vi "全局1.vi"() -> ()   [LabVIEW 2016, in "数据传输系统-05.lvlib"]
panel:
  out "2086上传":bool caption="2086"
  out "固件版本":T1
  out "版本信息":string
  out "系统信息":u16[](array[numeric]) caption="校准点信息"
  in  "告警信息":T2
  out "配置文件队列名":T3
  out "校准信息改变时间":string
  in  "采配水关键参数":cluster{"配水时间":dbl, "沉淀时间":dbl, "清洗时间":dbl}
  in  "CODCr校准信息":T4
  in  "总氮校准信息":T4
  in  "总磷校准信息":T4
  in  "氨氮校准信息":T4
  in  "CODMn校准信息":T4
  out "校准信息改变":T5
  out "关键参数改变":T6
  in  "CODCr关键参数":T7
  in  "总氮关键参数":T7
  in  "总磷关键参数":T7
  in  "氨氮关键参数":T7
  in  "CODMn关键参数":T7
  out "读取各参数测量周期的值":u16[](array[numeric]) caption="读取试剂余量的值"
  out "读取试剂余量的值":u16[](array[numeric])
  out "软件自动重启":dbl
  out "与工控软件通信":bool
  in  "QN":string
  in  "命令编码CN":string
  in  "数据":string
  out "数据发送起始时间":timestamp format="%<%.3X\n%Y/%m/%d>T"
  out "数据接收超时指示灯":bool
  out "实时小时数据上传":bool
  out "核查数据上传":bool
  out "反控数据":bool caption="超标留样"
  in  "table元素":string
  out "超标留样":bool
  out "测量周期":bool
  out "运行模式":bool
  out "系统状态":bool
  out "读取报文首页显示":string
  out "发送报文首页显示":string
  out "通讯包字符串":string
  out "数据输出":string
  out "register values":u16[](array[numeric]) caption="读取寄存器的值"
  out "系统编码ST":string="21"
  in  "枚举":enum16{"返回请求应答", "上传数据", "返回执行结果"}(ring)
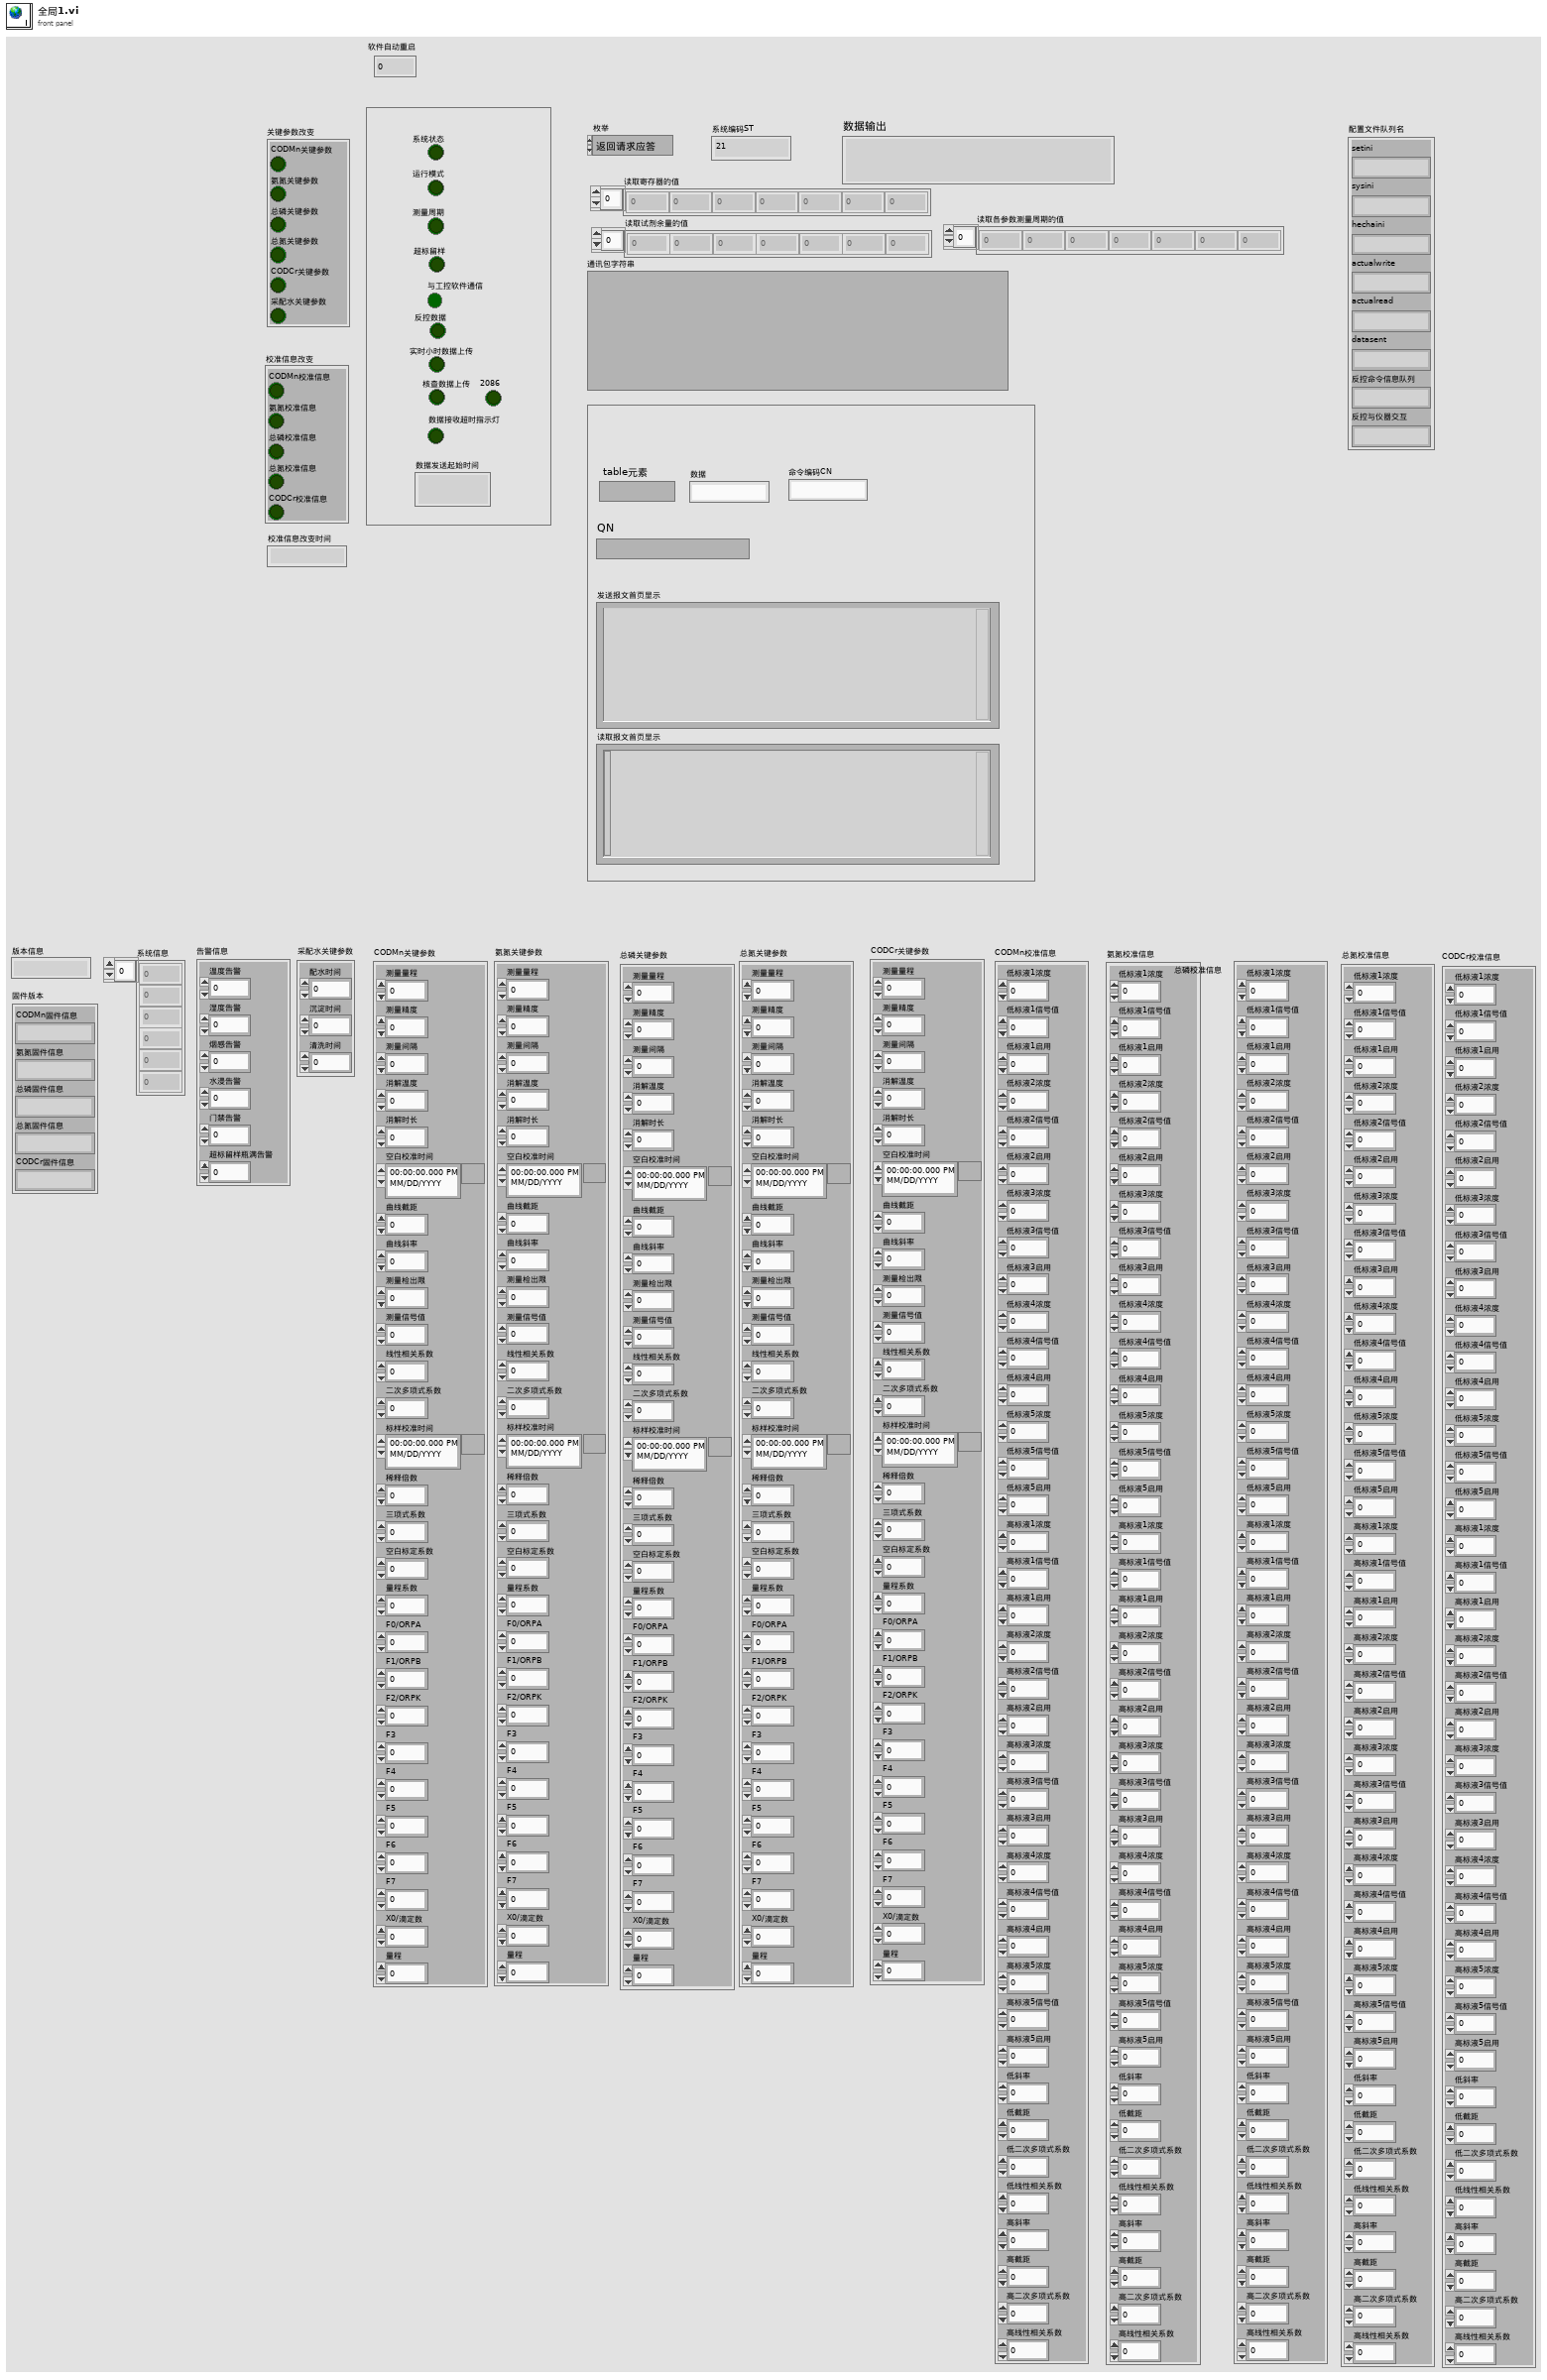
[diagram p1: front panel]
types:
  T1 = cluster{"CODMn固件信息":string, "氨氮固件信息":string, "总磷固件信息":string, "总氮固件信息":string, "CODCr固件信息":string}
  T2 = cluster{"温度告警":u16, "湿度告警":u16, "烟感告警":u16, "水浸告警":u16, "门禁告警":u16, "超标留样瓶满告警":u16}
  T3 = cluster{"setini":string, "sysini":string, "hechaini":string, "actualwrite":string, "actualread":string, "datasent":string, "反控命令信息队列":string, "反控与仪器交互":string}
  T4 = cluster{"低标液1浓度":dbl, "低标液1信号值":dbl, "低标液1启用":u16, "低标液2浓度":dbl, "低标液2信号值":dbl, "低标液2启用":u16, "低标液3浓度":dbl, "低标液3信号值":dbl, "低标液3启用":u16, "低标液4浓度":dbl, "低标液4信号值":dbl, "低标液4启用":u16, "低标液5浓度":dbl, "低标液5信号值":dbl, "低标液5启用":u16, "高标液1浓度":dbl, "高标液1信号值":dbl, "高标液1启用":u16, "高标液2浓度":dbl, "高标液2信号值":dbl, "高标液2启用":u16, "高标液3浓度":dbl, "高标液3信号值":dbl, "高标液3启用":u16, "高标液4浓度":dbl, "高标液4信号值":dbl, "高标液4启用":u16, "高标液5浓度":dbl, "高标液5信号值":dbl, "高标液5启用":u16, "低斜率":dbl, "低截距":dbl, "低二次多项式系数":dbl, "低线性相关系数":dbl, "高斜率":dbl, "高截距":dbl, "高二次多项式系数":dbl, "高线性相关系数":dbl}
  T5 = cluster{"CODMn校准信息":bool, "氨氮校准信息":bool, "总磷校准信息":bool, "总氮校准信息":bool, "CODCr校准信息":bool}
  T6 = cluster{"CODMn关键参数":bool, "氨氮关键参数":bool, "总磷关键参数":bool, "总氮关键参数":bool, "CODCr关键参数":bool, "采配水关键参数":bool}
  T7 = cluster{"测量量程":dbl, "测量精度":dbl, "测量间隔":dbl, "消解温度":dbl, "消解时长":dbl, "空白校准时间":timestamp, "曲线截距":dbl, "曲线斜率":dbl, "测量检出限":dbl, "测量信号值":dbl, "线性相关系数":dbl, "二次多项式系数":dbl, "标样校准时间":timestamp, "稀释倍数":dbl, "三项式系数":dbl, "空白标定系数":dbl, "量程系数":dbl, "F0/ORPA":dbl, "F1/ORPB":dbl, "F2/ORPK":dbl, "F3":dbl, "F4":dbl, "F5":dbl, "F6":dbl, "F7":dbl, "X0/滴定数":dbl, "量程":dbl}
diagram:
